vi "WildBugChilGru_V0.191.vi"() -> ()   [LabVIEW 2014]
uses:
  <vilib>/Utility/miscctls.llb/LVPointTypeDef.ctl
  <vilib>/Utility/xml.llb/Read From XML File(string).vi
  <vilib>/Utility/NIReport.llb/Append Report Text (str wrap).vi
  <vilib>/Utility/xml.llb/Write to XML File(string).vi
  <vilib>/Instr/_visa.llb/VISA Configure Serial Port (Instr).vi
  <vilib>/Analysis/3filter.llb/IIR Filter (DBL).vi
  <vilib>/Utility/NIReport.llb/NI_report.lvclass
  <vilib>/Analysis/NI_AALBase.lvlib
  <vilib>/gmath/NI_Gmath.lvlib
  <vilib>/Analysis/NI_AALPro.lvlib
panel:
  in  "Registerkarte":T1(tab)
  in  "Gleitender Mittelwert":u8=35
  in  "Differenzenquotient":u8=12
  in  "Polynom":u8=15
  in  "n vom Gas [1/min]":dbl=5000.0
  in  "Zündung [Imp/U]":u8=5
  in  "Übersetzung ermitteln aus":T2(ring)
  in  "Getriebe [1:]":dbl=5.343
  in  "Reifenumfang [m]":dbl=1.222
  in  "Dauer [s]":dbl=5.0
  in  "nKuWe/nRolle":dbl=10.0
  in  "Rolle [Inkr/U]":u16=10
  in  "Rollenumfang [m]":dbl=0.613
  in  "Rollenträgheit [kgm²]":dbl=0.402
  in  "Lufttemperatur [°C]":dbl=20.0
  in  "Luftfeuchtigkeit [%]":dbl=50.0
  in  "Luftdruck [mbar]":dbl=1013.0
  in  "Messung":bool
  in  "Ende":bool
  out "Datenspeicher":T3
  out "COM-Fehlerrate":string="0 / 0,0%"
  in  "Konfiguration:":bool
  in  "Speichern":bool
  in  "Drucken":bool
  out "Pmax":string="0,0 PS"
  out "Ergebnis":string="0,0 PS bei 0 1/min   |   0,0 Nm bei 0 1/min   |   vmax: 2147483647 km/h\nDIN 70020 k =1,000 (20 °C, 50 %, 1013 mbar)\n20.11.2016 20:05 "
  in  "Fahrzeugdaten":string="Hier die Fahrzeugdaten eingeben"
  out "XY-Graph":cluster{dbl[], dbl[]}[](graph)
  out "Untersetzung\nermittelt":bool
  out "Untersetzung":dbl format="%#.2f"
  in  "Start [F1]":bool
  out "Füllstand Lesepuffer":u64(slide) scale=1.0..100.0
  out "Hinterrad\n[km/h]":dbl(knob) scale=0.0..150.0
  out "Welle\n[1/min]":cluster{dbl, dbl}(knob) scale=0.0..12000.0
  out "Lesepuffer":string="\n"
  in  "Serielle Schnittstelle":refnum<visa-resource-name>="COM6"
  out "Untersetzung-Graph":dbl(graph)=2.6802446808510636 caption="Untersetzung"
  # "1. n konstant halten\n2. START\n3. n weiter halten\n4. bei GO: Vollgas\n5. vom Gas gehen"
  # "Zündung\nRolle"
  # "Untersetzung aus:"
  # "Eingabe <> Messen"
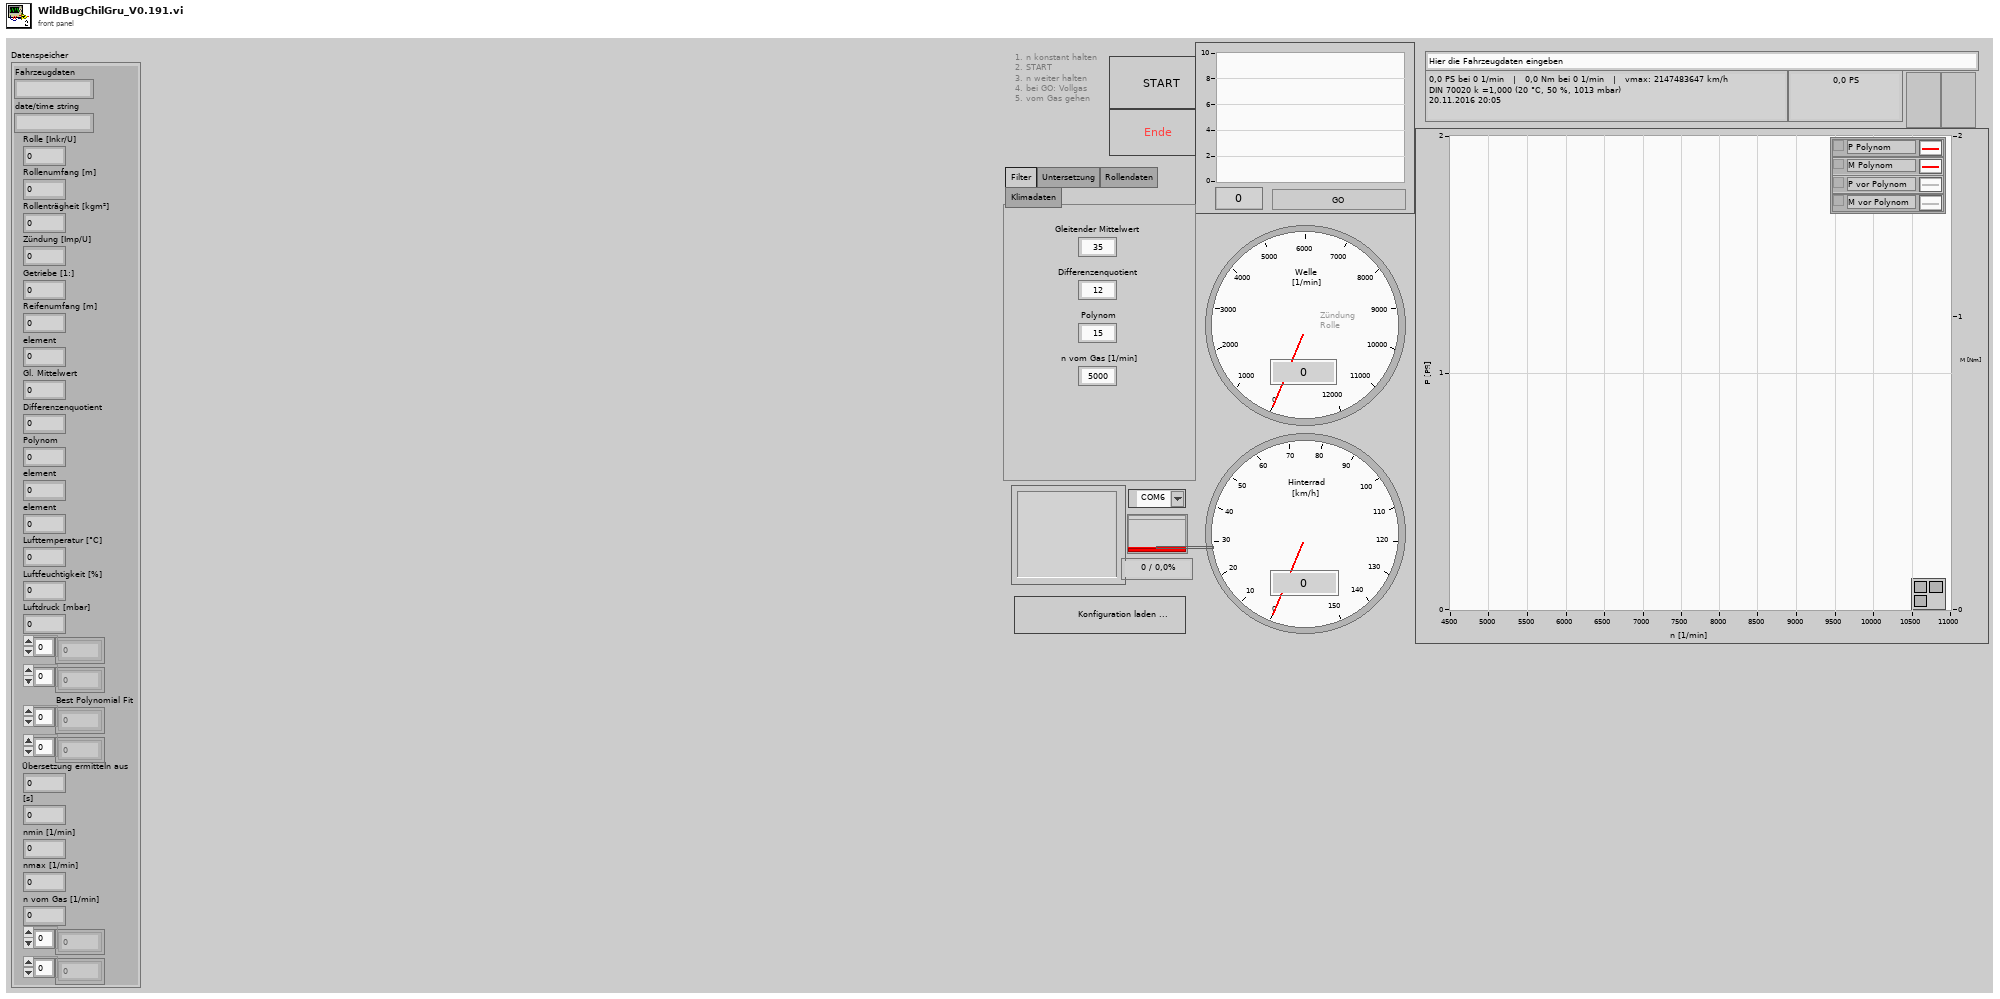
[diagram p1: front panel]
types:
  T1 = enum32{"Filter", "Untersetzung", "Rollendaten", "Klimadaten"}
  T2 = enum8{"Zündsignal", "Getriebe & Reifen", "nKuWe / nRolle"}
  T3 = cluster{"Fahrzeugdaten":string, "date/time string":string, "Rolle [Inkr/U]":u16, "Rollenumfang [m]":dbl, "Rollenträgheit [kgm²]":dbl, "Zündung [Imp/U]":u8, "Getriebe [1:]":dbl, "Reifenumfang [m] ":dbl, "element":dbl, "Gl. Mittelwert":u8, "Differenzenquotient":u8, "Polynom":u8, "element":dbl, "element":dbl, "Lufttemperatur [°C]":dbl, "Luftfeuchtigkeit [%]":dbl, "Luftdruck [mbar]":dbl, dbl[], dbl[], "Best Polynomial Fit":dbl[], dbl[], "Übersetzung ermitteln aus":u8, "[s]":dbl, "nmin [1/min]":dbl, "nmax [1/min]":dbl, "n vom Gas [1/min]":dbl, dbl[], i32[]}
  T4 = enum16{"Kleinste Quadrate", "Kleinestes absolutes Reiduum", "Biquadrat"}
  T5 = enum8{"Enabled", "Disabled", "Disabled and Grayed Out"}
  T6 = cluster{"Fahrzeugdaten":string, "date/time string":string, "Rolle [Inkr/U]":u16, "Rollenumfang [m]":dbl, "Rollenträgheit [kgm²]":dbl, "Zündung [Imp/U]":u8, "Getriebe [1:]":dbl, "Reifenumfang [m] ":dbl, "mean value":dbl, "Gleitender Mittelwert":u8, "Differenzenquotient":u8, "Polynom":u8, dbl, "element":dbl, "Lufttemperatur [°C]":dbl, "Luftfeuchtigkeit [%]":dbl, "Luftdruck [mbar]":dbl, dbl[], dbl[], "Best Polynomial Fit":dbl[], dbl[], "Übersetzung ermitteln aus":enum8{"Zündsignal", "Getriebe & Reifen", "nKuWe / nRolle"}, "Dauer [s]":dbl, dbl, dbl, "n vom Gas [1/min]":dbl, dbl[], i32[]}
  T7 = typedef "LVPointTypeDef.ctl" = cluster{"Horizontal":i16, "Vertical":i16}
  T8 = cluster{string, string, u16, dbl, dbl, u8, dbl, dbl, dbl, u8, u8, u8, dbl, dbl, dbl, dbl, dbl, dbl[], dbl[], dbl[], dbl[], i32, dbl, dbl, dbl, dbl, dbl[], i32[]}
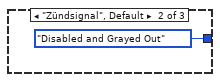
[diagram p2: hidden frame]
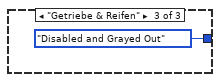
[diagram p3: hidden frame]
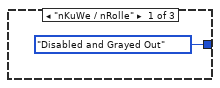
[diagram p4: hidden frame]
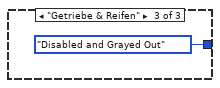
[diagram p5: hidden frame]
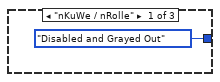
[diagram p6: hidden frame]
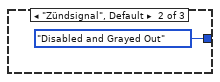
[diagram p7: hidden frame]
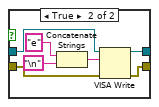
[diagram p11: hidden frame]
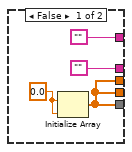
[diagram p13: hidden frame]
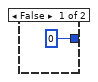
[diagram p14: hidden frame]
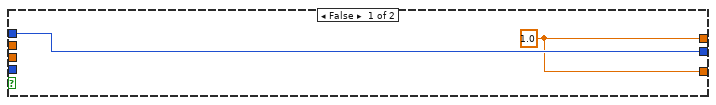
[diagram p16: hidden frame]
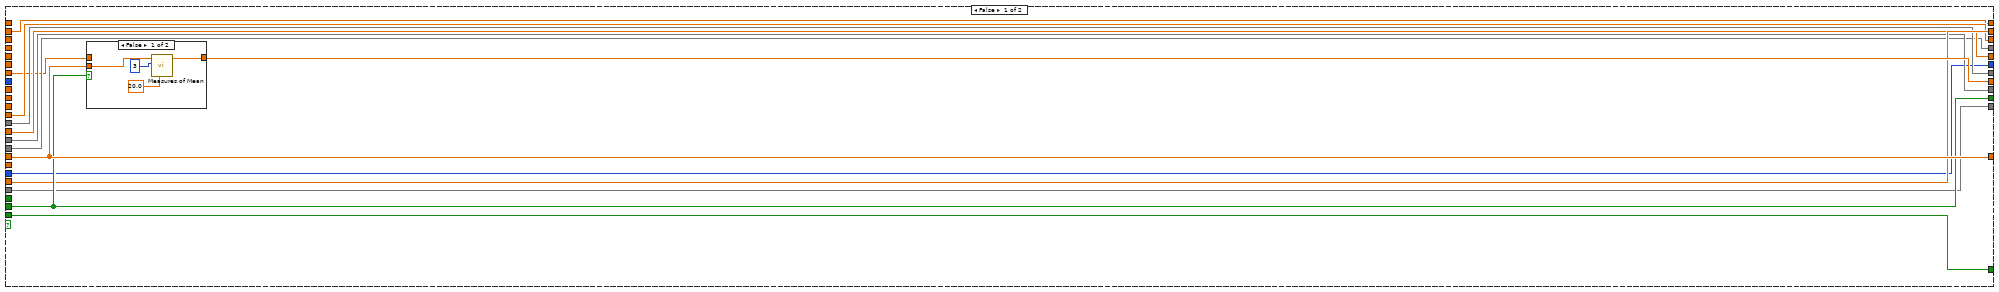
[diagram p17: hidden frame]
diagram:
  n1 = while {
    stop <- w1 stop-if-true
    n2 = event shown="[0] \"Start [F1]\": Wertänderung" {
      selector: _ -> [_ _]
      dyn-events: _ -> [_ _]
      timeout: _ -> [_ _]
      tunnel: [_ TRUE] -> w1
      event "Start [F1]": Value Change {
        n3 = event-data() -> ("NewVal"=w2:bool)  [unwired: 1 in, 5 out]
        n4 = case shown="True" w2 {
          frame False {
          }
          frame True {
            n5 = flat-sequence {
              tunnel: [w132] -> w117
              tunnel: [w131] -> w116
              tunnel: ["Messung"] -> w115
              tunnel: w117 -> [w145]
              tunnel: w116 -> [w144]
              tunnel: [0] -> w114
              tunnel: [1.0 ("element")] -> w113
              tunnel: [w142] -> w112
              tunnel: [w156] -> w111
              tunnel: [0] -> w110
              tunnel: [w142] -> w109
              tunnel: [-5] -> w108
              tunnel: [w153] -> w107
              tunnel: [w151] -> w106
              tunnel: [w150] -> w105
              tunnel: [0.0] -> w104
              tunnel: [w145] -> w103
              tunnel: [w144] -> w102
              tunnel: w115 -> [w143]
              tunnel: [w143] -> w101
              tunnel: w114 -> [w180]
              tunnel: [w180] -> w100
              tunnel: w113 -> [w179]
              tunnel: [w179] -> w99
              tunnel: w112 -> [w178]
              tunnel: [w178] -> w98
              tunnel: w111 -> [w177]
              tunnel: [w177] -> w97
              tunnel: w110 -> [w176]
              tunnel: [w176] -> w96
              tunnel: w109 -> [w175]
              tunnel: [w175] -> w95
              tunnel: w108 -> [w174]
              tunnel: [w174] -> w94
              tunnel: w107 -> [w173]
              tunnel: [w173] -> w93
              tunnel: w106 -> [w172]
              tunnel: [w172] -> w92
              tunnel: w105 -> [w171]
              tunnel: [w171] -> w91
              tunnel: w104 -> [w170]
              tunnel: [w170] -> w90
              tunnel: w103 -> [w169]
              tunnel: [w166] -> w89
              tunnel: w102 -> [w168]
              tunnel: [w167] -> w88
              tunnel: [w165] -> w87
              tunnel: w101 -> [w165]
              tunnel: w100 -> [w204]
              tunnel: [w204] -> w86
              tunnel: w99 -> [w203]
              tunnel: [w203] -> w85
              tunnel: w98 -> [w202]
              tunnel: [w202] -> w84
              tunnel: w97 -> [w201]
              tunnel: [w201] -> w83
              tunnel: w96 -> [w200]
              tunnel: [w200] -> w82
              tunnel: w95 -> [w199]
              tunnel: [w199] -> w81
              tunnel: w94 -> [w198]
              tunnel: [w198] -> w80
              tunnel: w93 -> [w197]
              tunnel: [w197] -> w79
              tunnel: w92 -> [w196]
              tunnel: [w196] -> w78
              tunnel: w91 -> [w195]
              tunnel: [w195] -> w77
              tunnel: w90 -> [w194]
              tunnel: [w194] -> w76
              tunnel: w89 -> [w193]
              tunnel: [w193] -> w75
              tunnel: w88 -> [w192]
              tunnel: [w192] -> w74
              tunnel: w87 -> [w190]
              tunnel: [w190] -> w73
              tunnel: w86 -> [w220]
              tunnel: [w220] -> w72
              tunnel: w85 -> [w219]
              tunnel: [w219] -> w71
              tunnel: w84 -> [w218]
              tunnel: [w218] -> w70
              tunnel: w83 -> [w217]
              tunnel: [w217] -> w69
              tunnel: w82 -> [w216]
              tunnel: [w216] -> w68
              tunnel: w81 -> [w215]
              tunnel: [w215] -> w67
              tunnel: w80 -> [w214]
              tunnel: [w214] -> w66
              tunnel: w79 -> [w213]
              tunnel: [w213] -> w65
              tunnel: w78 -> [w212]
              tunnel: [w212] -> w64
              tunnel: w77 -> [w211]
              tunnel: [w211] -> w63
              tunnel: w76 -> [w210]
              tunnel: [w210] -> w62
              tunnel: w75 -> [w209]
              tunnel: [w208] -> w61
              tunnel: w74 -> [w206]
              tunnel: [w207] -> w60
              tunnel: w73 -> [w205]
              tunnel: w72 -> [w293]
              tunnel: w71 -> [w292]
              tunnel: w70 -> [w291]
              tunnel: w69 -> [w290]
              tunnel: w68 -> [w289]
              tunnel: w67 -> [w288]
              tunnel: w66 -> [w287]
              tunnel: w65 -> [w286]
              tunnel: w64 -> [w285]
              tunnel: w63 -> [w284]
              tunnel: w62 -> [w283]
              tunnel: w61 -> [w248]
              tunnel: [w293] -> w59
              tunnel: [w292] -> w58
              tunnel: [w291] -> w57
              tunnel: [w290] -> w56
              tunnel: [w289] -> w55
              tunnel: [w288] -> w54
              tunnel: [w287] -> w53
              tunnel: [w286] -> w52
              tunnel: [w285] -> w51
              tunnel: [w284] -> w50
              tunnel: [w283] -> w49
              tunnel: [w248] -> w48
              tunnel: [w247] -> w47
              tunnel: [w282] -> w46
              tunnel: [w281] -> w45
              tunnel: [w280] -> w44
              tunnel: ["Gleitender Mittelwert"] -> w43
              tunnel: w60 -> [w247]
              tunnel: [w302] -> w9
              tunnel: [w303] -> w10
              tunnel: [w304] -> w11
              tunnel: [w305] -> w12
              tunnel: [w296] -> w7
              tunnel: [w295] -> w8
              tunnel: [w306] -> w13
              tunnel: [w307] -> w14
              tunnel: [w308] -> w16
              tunnel: [w309] -> w18
              tunnel: [w310] -> w19
              tunnel: [w311] -> w20
              tunnel: [w312] -> w37
              tunnel: [w313] -> w39
              tunnel: [w314] -> w40
              tunnel: [w315] -> w41
              tunnel: [w316] -> w42
              tunnel: w59 -> [w316]
              tunnel: w58 -> [w315]
              tunnel: w57 -> [w314]
              tunnel: w56 -> [w313]
              tunnel: w55 -> [w312]
              tunnel: w54 -> [w311]
              tunnel: w53 -> [w310]
              tunnel: w52 -> [w309]
              tunnel: w51 -> [w308]
              tunnel: w50 -> [w307]
              tunnel: w49 -> [w306]
              tunnel: w48 -> [w298]
              tunnel: w47 -> [w297]
              tunnel: w46 -> [w305]
              tunnel: w45 -> [w304]
              tunnel: w44 -> [w303]
              tunnel: w43 -> [w302]
              frame #0 {
                w137 = u16 0 items=["None", "XON/XOFF", "RTS/CTS", "XON/XOFF & RTS/CTS", "DTR/DSR", "XON/XOFF & DTR/DSR"] ("flow control (0:none)")
                w138 = u16 10 items=["1.0"=10, "1.5"=15, "2.0"=20] ("stop bits (10: 1 bit)")
                w130 = FALSE  # Enable Termination Char (T)
                w133 = u32 10000  # timeout (10sec)
                n6 = call-poly "VISA Configure Serial Port"("VISA resource name"="Serielle Schnittstelle", "timeout (10sec)"=w133, "Enable Termination\nChar (T)"=w130, "baud rate (9600)"=u32 250000 ("baudrate (250000)"), "data bits (8)"=u16 8, "parity (0:none)"=enum16{"None", "Odd", "Even", "Mark", "Space"}."None", "stop bits (10: 1 bit)"=w138, "flow control (0:none)"=w137) -> ("VISA resource name out"=w135:refnum<visa-resource-name>, "error out"=w134:errorcluster)  [unwired: 6 in]
                n7 = VISA Clear(VISA resource name=w135, error in (no error)=w134) -> (VISA resource name out=w132:refnum<visa-resource-name>, error out=w131:errorcluster)
              }
              frame #1 {
                w146 = T5."Disabled and Grayed Out" ("Deaktiviert")
                w149 = 0.0  # Graphen löschen
                w152 = 0
                w157 = 0.0
                w142 = FALSE
                w150 = ""
                n8 = case shown="True" w143 {
                  frame False {
                  }
                  frame True {
                    n9 = Wait (ms)(milliseconds to wait=u32 2000 ("Zu wartende ms")) -> ()  [unwired: 1 out]
                    n10 = property on="Untersetzung\nermittelt" class="Bool. (strikt)"("Blinking"=TRUE ("Blinkend"), "BoolText.Text"="Lese Klimadaten" ("Beschriftung.Text")) -> ()  [unwired: 2 in, 2 out]
                  }
                }
                n11 = Build Array(w149) -> (w148:dbl[])
                n12 = property on="Drucken" class="Bool. (strikt)"("DisabledEnum"=w146) -> ()  [unwired: 2 in, 2 out]
                n13 = property on="Übersetzung ermitteln aus" class="Enum (strikt)"("DisabledEnum"=w146) -> ()  [unwired: 2 in, 2 out]
                n14 = property on="Konfiguration:" class="Bool. (strikt)"("DisabledEnum"=w146) -> ()  [unwired: 2 in, 2 out]
                n15 = property on="Ende" class="Bool. (strikt)"("DisabledEnum"=w146) -> ()  [unwired: 2 in, 2 out]
                n16 = property on="Speichern" class="Bool. (strikt)"("DisabledEnum"=w146) -> ()  [unwired: 2 in, 2 out]
                n17 = local write "Pmax"(w150) -> ()
                n18 = property on="Untersetzung-Graph" class="SVDiagr (strikt)"("History Data"=w148) -> ()  [unwired: 2 in, 2 out]
                n19 = local write "COM-Fehlerrate"(w150) -> ()
                n20 = local write "Ergebnis"(w150) -> ()
                n21 = Initialize Array(0.0 ("y"), 0) -> (w153:dbl[])
                n22 = Initialize Array(w152, w152) -> (w151:i32[])
                n23 = Initialize Array(w157, w157) -> (w156:dbl[])
              }
              frame #2 {
                n24 = case shown="False" w165 {
                  tunnel: w169 -> [w182 w186]
                  tunnel: w168 -> [w181 w185]
                  tunnel: [w181 w184] -> w167
                  tunnel: [w182 w183] -> w166
                  frame False {
                  }
                  frame True {
                    n25 = Concatenate Strings("e" ("String"), "\n") -> (w189:string)
                    n26 = VISA Write(VISA resource name=w186, write buffer=w189, error in (no error)=w185) -> (VISA resource name out=w183:refnum<visa-resource-name>, error out=w184:errorcluster)  [unwired: 1 out]
                  }
                }
              }
              frame #3 {
                n27 = Wait (ms)(milliseconds to wait=u32 500 ("Zu wartende ms")) -> ()  [unwired: 1 out]
              }
              frame #4 {
                n28 = case shown="True" w205 {
                  tunnel: w209 -> [w222 w242]
                  tunnel: [w222 w241] -> w208
                  tunnel: [w221 w240] -> w207
                  tunnel: w206 -> [w221 w239]
                  frame False {
                  }
                  frame True {
                    w224 = ";" ("Regulärer Ausdruck")
                    n29 = property class="Instr"(reference=w242, error in=w239) -> (reference out=w245:refnum<visa-resource-name>, error out=w244:errorcluster, "Serial Settings:Number of Bytes at Serial Port"=w243:u32)
                    n30 = VISA Read(VISA resource name=w245, byte count=w243, error in (no error)=w244) -> (VISA resource name out=w241:refnum<visa-resource-name>, read buffer=w236:string, error out=w240:errorcluster)  [unwired: 1 out]
                    n31 = Search and Replace String(replace all?=TRUE ("Alle ersetzen? (F)"), input string=w236, search string="." ("Such-String"), replace string="," ("Ersetzungs-String (\"\")")) -> (result string=w229:string)  [unwired: 4 in, 3 out]
                    n32 = Match Pattern(string=w229, regular expression=w224) -> (before substring=w227:string, after substring=w228:string)  [unwired: 1 in, 2 out]
                    n33 = Fract/Exp String To Number(string=w227) -> (number=w235:dbl)  [unwired: 3 in, 1 out]
                    n34 = Match Pattern(string=w228, regular expression=w224) -> (before substring=w226:string, after substring=w225:string)  [unwired: 1 in, 2 out]
                    n35 = local write "Lufttemperatur [°C]"(w235) -> ()
                    n36 = Fract/Exp String To Number(string=w226) -> (number=w232:dbl)  [unwired: 3 in, 1 out]
                    n37 = Match Pattern(string=w225, regular expression=w224) -> (before substring=w223:string)  [unwired: 1 in, 3 out]
                    n38 = Fract/Exp String To Number(string=w223) -> (number=w234:dbl)  [unwired: 3 in, 1 out]
                    n39 = Divide(x=w232, y=100.0 ("x")) -> (x/y=w233:dbl)
                    n40 = local write "Luftdruck [mbar]"(w233) -> ()
                    n41 = local write "Luftfeuchtigkeit [%]"(w234) -> ()
                  }
                }
              }
              frame #5 {
                n42 = Wait (ms)(milliseconds to wait=u32 2000 ("Zu wartende ms")) -> ()  [unwired: 1 out]
                n43 = Add(x="Lufttemperatur [°C]", y=273.15) -> (x+y=w263:dbl)
                n44 = Divide ("M_Welle [Nm]")(x=300.0, y=w263) -> (x/y=w266:dbl)
                n45 = Multiply(x="Luftfeuchtigkeit [%]", y=0.01) -> (x*y=w277:dbl)
                n46 = Divide ("M_Welle [Nm]")(x=w263, y=293.15) -> (x/y=w261:dbl)
                n47 = Multiply(x=w277, y=240800000000.0) -> (x*y=w251:dbl)
                n48 = Power Of X(1:w266, 2:5.0) -> (0:w264:dbl)
                n49 = Multiply(x=w251, y=w264) -> (x*y=w271:dbl)
                n50 = Multiply(x=w266, y=-22.644) -> (x*y=w272:dbl)
                n51 = Power Of X(1:w261, 2:0.5) -> (0:w258:dbl)
                n52 = Exponential(1:w272) -> (0:w270:dbl)
                n53 = Multiply(x=w271, y=w270) -> (x*y=w269:dbl)
                n54 = Subtract "p_Trocken [mbar]"(x="Luftdruck [mbar]", y=w269) -> (x-y=w267:dbl)
                n55 = Divide ("M_Welle [Nm]")(x=1013.0, y=w267) -> (x/y=w259:dbl)
                n56 = Multiply "Korrekturfaktor DIN 70020"(x=w259, y=w258) -> (x*y=w282:dbl)
                n57 = Divide(x="Gleitender Mittelwert", y=2) -> (x/y=w255:dbl)
                n58 = Round Toward -Infinity(1:w255) -> (0:w254:dbl)
                n59 = call <vilib>:"Smoothing Filter Coefficients.vi"("shape"=1, "half-width"=w254, "type"=0) -> ("forward coefficients"=w280:dbl[], "reverse coefficients"=w281:dbl[])  [unwired: 6 in, 1 out]
              }
              frame #6 {
                n60 = Concatenate Strings("m" ("String"), "\n") -> (w301:string)
                n61 = property on="Untersetzung\nermittelt" class="Bool. (strikt)"("Blinking"=FALSE ("Blinkend")) -> ()  [unwired: 2 in, 2 out]
                n62 = VISA Write(VISA resource name=w298, write buffer=w301, error in (no error)=w297) -> (VISA resource name out=w295:refnum<visa-resource-name>, error out=w296:errorcluster)  [unwired: 1 out]
              }
            }
            n63 = while {
              tunnel: w8 -> [w447]
              tunnel: w7 -> [w446]
              shift-right: [w517] -> _
              shift-left: w14 -> [w462]
              shift-right: [w512] -> _
              shift-left: w13 -> [w516]
              shift-right: [w511] -> _
              shift-left: w13 -> [w515]
              shift-right: [w466] -> _
              shift-left: w13 -> [w514]
              shift-right: [w493] -> _
              shift-left: w42 -> [w513]
              shift-right: [w454] -> w25
              shift-left: w41 -> [_]
              shift-right: [w472] -> w29
              shift-left: w13 -> [w494]
              shift-right: [w504] -> w27
              shift-left: w13 -> [w468]
              shift-right: [w467] -> _
              shift-left: w18 -> [w508]
              shift-right: [w505] -> _
              shift-left: w40 -> [w482]
              shift-right: [w448] -> _
              shift-left: w39 -> [_]
              shift-right: [w453] -> _
              shift-left: w39 -> [_]
              shift-right: [w503] -> w28
              shift-left: w39 -> [w501]
              shift-right: [w502] -> _
              shift-left: w39 -> [w500]
              shift-right: [w488] -> w36
              shift-left: w18 -> [w499]
              shift-right: [w492] -> _
              shift-left: w18 -> [w497]
              shift-right: [w491] -> w32
              shift-left: w18 -> [w498]
              shift-right: [w490] -> w35
              shift-left: w18 -> [w496]
              shift-right: [w489] -> w34
              shift-left: w18 -> [w495]
              tunnel: [w487] -> w38
              shift-right: [w483] -> w33
              shift-left: w37 -> [w485]
              tunnel: [w486] -> w3
              tunnel: ["n vom Gas [1/min]"] -> w31
              tunnel: ["Rollenumfang [m]"] -> w30
              tunnel: ["Rollenumfang [m]"] -> w24
              shift-right: [w479] -> _
              shift-left: w20 -> [w445]
              shift-right: [w473] -> _
              shift-left: w19 -> [w478]
              shift-right: [w474] -> _
              shift-left: w13 -> [w477]
              shift-right: [w475] -> _
              shift-left: w13 -> [w476]
              shift-right: [w471] -> w17
              shift-left: w18 -> [w470]
              shift-right: [w465] -> _
              shift-left: _ -> [w464]
              shift-right: [w469] -> w15
              shift-left: w16 -> [w463]
              tunnel: [w461] -> w4
              tunnel: w12 -> [w454]
              tunnel: w11 -> [w448]
              tunnel: w10 -> [w453]
              tunnel: w9 -> [w452]
              stop <- w487 stop-if-true
              n64 = property class="Instr"(reference=w447, error in=w446) -> (reference out=w457:refnum<visa-resource-name>, error out=w456:errorcluster, "Serial Settings:Number of Bytes at Serial Port"=w459:u32)
              n65 = Greater?(x=w459, y=u32 1 ("min. Bytes")) -> (0:w455:bool)
              n66 = case shown="True" w455 {
                tunnel: w459 -> [_ w519]
                tunnel: [u32 0 ("Bytes at Port") w519] -> w458
                frame False {
                }
                frame True {
                }
              }
              n67 = case shown="1.." w458 {
                selector: w458 -> [_ w772]
                tunnel: [w722 w766] -> w486
                tunnel: [w721 w767] -> w461
                tunnel: [w726 w768] -> w511
                tunnel: [w727 w765] -> w512
                tunnel: w462 -> [w728 w763]
                tunnel: [w728 w761] -> w517
                tunnel: w516 -> [w727 w753]
                tunnel: w515 -> [w726 w752]
                tunnel: [w723 w751] -> w466
                tunnel: w514 -> [w723 w750]
                tunnel: w513 -> [w725 _]
                tunnel: [w725 w733] -> w493
                tunnel: [w724 w739] -> w465
                tunnel: w464 -> [w724 w738]
                tunnel: w457 -> [w721 w730]
                tunnel: w456 -> [w722 w729]
                frame 0, Default {
                  # "No data in from serial port - Nothing to do."
                }
                frame 1.. {
                  # "Hz Drum"
                  n68 = VISA Read(VISA resource name=w730, byte count=w772, error in (no error)=w729) -> (VISA resource name out=w767:refnum<visa-resource-name>, read buffer=w764:string, error out=w766:errorcluster)  [unwired: 1 out]
                  n69 = Concatenate Strings(w763, w764) -> (w735:string)
                  "Lesepuffer" <- w735
                  n70 = Spreadsheet String To Array(delimiter (Tab)="\n" ("regular expression"), format string="%s" ("regular expression"), spreadsheet string=w735, array type (2D Dbl)=string[] [] ("Array 2")) -> (array=w744:string[])
                  n71 = Match Pattern(string=w735, regular expression="[\\n]") -> (before substring=w742:string, after substring=w762:string, offset past match=w776:i32)  [unwired: 1 in, 1 out]
                  n72 = Array Size(array=w744) -> (size(s)=w748:i32)
                  n73 = Match Pattern(string=w742, regular expression="[;]") -> (before substring=w740:string, after substring=w741:string, offset past match=w737:i32)  [unwired: 1 in, 1 out]
                  n74 = Subtract "aktuelle Zeilenanzahl"(x=w748, y=1) -> (x-y=w733:i32)
                  n75 = property on="Füllstand Lesepuffer" class="Schieber (strikt)"() -> ("Scale.Maximum"=w732:dbl)  [unwired: 2 in, 2 out]
                  n76 = Match Pattern(string=w741, regular expression="[;]") -> (before substring=w771:string, after substring=w774:string, offset past match=w759:i32)  [unwired: 1 in, 1 out]
                  n77 = Match Pattern(string=w774, regular expression="[;]") -> (before substring=w770:string, after substring=w769:string, offset past match=w757:i32)  [unwired: 1 in, 1 out]
                  n78 = Greater Or Equal To 0?(x=w737) -> (x >= 0?=w736:bool)
                  n79 = Greater?(x=w733, y=w732) -> (0:w734:bool)
                  n80 = Greater Or Equal To 0?(x=w757) -> (x >= 0?=w756:bool)
                  n81 = Greater Or Equal To 0?(x=w759) -> (x >= 0?=w758:bool)
                  n82 = Greater Or Equal To 0?(x=w776) -> (x >= 0?=w760:bool)
                  n83 = Select(t=w733, s=w734, f=w732) -> (s? t:f=w731:dbl)
                  n84 = Build Array(w760, w758, w736, w756) -> (w755:bool[])
                  n85 = property on="Füllstand Lesepuffer" class="Schieber (strikt)"("Scale.Maximum"=w731) -> ()  [unwired: 2 in, 2 out]
                  n86 = And Array Elements(Boolean array=w755) -> (logical AND=w754:bool)
                  n87 = case shown="True" w754 {
                    tunnel: w771 -> [_ w787]
                    tunnel: w770 -> [_ w792]
                    tunnel: w769 -> [_ w791]
                    tunnel: [w780 w790] -> w768
                    tunnel: [w781 w789] -> w765
                    tunnel: w762 -> [_ w788]
                    tunnel: [w782 w788] -> w761
                    tunnel: w735 -> [w782 _]
                    tunnel: w753 -> [w781 _]
                    tunnel: w752 -> [w780 _]
                    tunnel: [w779 w786] -> w751
                    tunnel: w750 -> [w779 _]
                    tunnel: w740 -> [_ w785]
                    tunnel: [w778 w783] -> w739
                    tunnel: w738 -> [w778 _]
                    frame False {
                    }
                    frame True {
                      # "Cyclecounter"
                      # "Hz ComLevel"
                      # "ComLevel\nLevel 10 =   6Hz \nLevel 5 =   12Hz \nLevel 4 =   15Hz\nLevel 3 =   20Hz\nLevel 2 =   33Hz\nLevel 1 =   62Hz"
                      # "Hz Drum"
                      # "Hz Engine"
                      # "t4m"
                      n88 = Fract/Exp String To Number(string=w785) -> (number=w784:dbl)  [unwired: 3 in, 1 out]
                      n89 = Fract/Exp String To Number(string=w791) -> (number=w790:dbl)  [unwired: 3 in, 1 out]
                      n90 = Fract/Exp String To Number(string=w787) -> (number=w786:dbl)  [unwired: 3 in, 1 out]
                      n91 = To Long Integer(number=w784) -> (32bit integer=w783:i32)
                      n92 = Fract/Exp String To Number(string=w792) -> (number=w789:dbl)  [unwired: 3 in, 1 out]
                    }
                  }
                }
              }
              "Füllstand Lesepuffer" <- w493
              n93 = Not Equal?(x=w464, y=w465) -> (x != y?=w449:bool)
              n94 = case shown="True" w449 {
                tunnel: w478 -> [w523 w534]
                tunnel: [w523 w546] -> w473
                tunnel: w477 -> [w522 w545]
                tunnel: [w522 w531] -> w474
                tunnel: w476 -> [w521 w544]
                tunnel: [w521 w532] -> w475
                tunnel: w465 -> [_ w530]
                tunnel: w463 -> [w520 w529]
                tunnel: [w520 w533] -> w469
                frame False {
                }
                frame True {
                  n95 = Build Array (concatenate)(w529, w530) -> (w533:i32[])
                  n96 = Greater Or Equal To 0?(x=w534) -> (x >= 0?=w535:bool)
                  n97 = case shown="True" w535 {
                    tunnel: [w547 w558] -> w531
                    tunnel: [w547 w559] -> w532
                    tunnel: [w548 w550] -> w546
                    tunnel: w545 -> [_ w552]
                    tunnel: w544 -> [_ w560]
                    tunnel: w530 -> [w548 w549]
                    tunnel: w534 -> [_ w550]
                    frame False {
                      w547 = 1.0
                    }
                    frame True {
                      w556 = 65536.0
                      n98 = Add(x=w550, y=w552) -> (x+y=w551:dbl)
                      n99 = Divide(x=w551, y=w556) -> (x/y=w561:dbl)
                      n100 = Increment(x=w560) -> (x+1=w559:dbl)
                      n101 = Round Toward -Infinity(1:w561) -> (0:w557:dbl)
                      n102 = Multiply(x=w557, y=w556) -> (x*y=w555:dbl)
                      n103 = Add(x=w555, y=w549) -> (x+y=w554:dbl)
                      n104 = Increment(x=w554) -> (x+1=w553:dbl)
                      n105 = Subtract(x=w553, y=w550) -> (x-y=w558:dbl)
                    }
                  }
                  n106 = Subtract(x=w531, y=w532) -> (x-y=w526:dbl)
                  n107 = Decrement(x=w526) -> (x-1=w525:dbl)
                  n108 = Max & Min(x=0, y=w525) -> (max(x,y)=w524:dbl)  [unwired: 1 out]
                  n109 = Divide(x=w524, y=w531) -> (x/y=w538:dbl)
                  n110 = Greater Than 0?(x=w524) -> (x > 0?=w528:bool)
                  n111 = Select(t=u32 16711680, s=w528, f=u32 0) -> (s? t:f=w539:u32)
                  n112 = Multiply(x=w538, y=100.0) -> (x*y=w536:dbl)
                  n113 = Format Into String(format string="%d / %.1f%%" ("Format-String"), w524, w536) -> (resulting string=→"COM-Fehlerrate":string)  [unwired: 2 in, 1 out]
                  n114 = property on="COM-Fehlerrate" class="Str"("Text.TextColor"=w539) -> ()  [unwired: 2 in, 2 out]
                }
              }
              n115 = case "Case-Struktur" shown="True" w449 {
                tunnel: w512 -> [w702 w713]
                tunnel: w511 -> [w701 w712]
                tunnel: [w702 w711] -> w510
                tunnel: [w701 w710] -> w509
                tunnel: w466 -> [_ w704]
                tunnel: w494 -> [w700 _]
                tunnel: [w700 w703] -> w472
                tunnel: w468 -> [_ w709]
                tunnel: "Rollenumfang [m]" -> [_ w708]
                frame False {
                }
                frame True {
                  w720 = 60.0 ("y")
                  n116 = Reciprocal "Abtastzeit [s]"(x=w704) -> (1/x=w703:dbl)
                  n117 = Divide "R [1/s]"(x=w712, y="Rolle [Inkr/U]") -> (x/y=w719:dbl)
                  n118 = Multiply "nR [1/min]"(x=w720, y=w719) -> (x*y=w710:dbl)
                  n119 = Divide(x=w713, y="Zündung [Imp/U]") -> (x/y=w716:dbl)
                  n120 = Multiply "nZ gemessen [1/min]"(x=w716, y=w720) -> (x*y=w711:dbl)
                  n121 = Multiply "nZ berechnet [1/min]"(x=w710, y=w709) -> (x*y=w718:dbl)
                  n122 = Multiply "[m/min]"(x=w710, y=w708) -> (x*y=w714:dbl)
                  n123 = Multiply "[km/h]"(x=w714, y=0.06) -> (x*y=→"Hinterrad\n[km/h]":dbl)
                  n124 = Bundle(w711, w718) -> (→"Welle\n[1/min]":cluster{dbl, dbl})  [unwired: 1 in]
                }
              }
              n125 = case shown="True" w449 {
                tunnel: w510 -> [_ w631]
                tunnel: w509 -> [_ w630]
                tunnel: "Rollenumfang [m]" -> [_ w634]
                tunnel: [w573 w600] -> w504
                tunnel: w468 -> [w562 w600]
                tunnel: w482 -> [w574 w638]
                tunnel: w508 -> [w575 w637]
                tunnel: [w574 w591] -> w505
                tunnel: [w575 w636] -> w467
                tunnel: w448 -> [_ w633]
                tunnel: w453 -> [_ w632]
                tunnel: [w572 w586] -> w503
                tunnel: [w571 w584] -> w502
                tunnel: w501 -> [w572 w629]
                tunnel: w500 -> [w571 _]
                tunnel: w452 -> [_ w582]
                tunnel: [w570 w606] -> w488
                tunnel: w499 -> [w570 _]
                tunnel: [w569 w621] -> w492
                tunnel: w497 -> [w569 _]
                tunnel: w494 -> [_ w619]
                tunnel: [w568 w607] -> w491
                tunnel: w498 -> [w568 _]
                tunnel: [w567 w623] -> w490
                tunnel: w496 -> [w567 _]
                tunnel: [w566 w622] -> w489
                tunnel: w495 -> [w566 _]
                tunnel: w454 -> [_ w611]
                tunnel: w485 -> [w565 w605]
                tunnel: "n vom Gas [1/min]" -> [_ w593]
                tunnel: [w565 w604] -> w483
                tunnel: w482 -> [_ w603]
                tunnel: w445 -> [w564 w599]
                tunnel: [w564 w598] -> w479
                tunnel: w472 -> [_ w597]
                tunnel: [w563 w596] -> w471
                tunnel: w470 -> [w563 w595]
                frame False {
                  n126 = case shown="False" w574 {
                    tunnel: w575 -> [w579 _]
                    tunnel: [w578 w580] -> w573
                    tunnel: w562 -> [_ w580]
                    frame False {
                      n127 = call <vilib>:"Measures of Mean.vi"("percent (trim)"=20.0, "type"=3, "x array"=w579) -> ("mean value"=w578:dbl)  [unwired: 7 in, 1 out]
                    }
                    frame True {
                    }
                  }
                }
                frame True {
                  w614 = 0.00135962  # [W] in [PS]
                  w625 = 0.10471975511965978  # 2*Pi/60
                  n128 = Build Array (concatenate) "akt. dT in Array einfügen"(w595, w597) -> (w596:dbl[])
                  n129 = Build Array (concatenate) "akt. Rollendrehzahl\nin Array einfügen"(w629, w630) -> (w586:dbl[])
                  n130 = local read "Übersetzung ermitteln aus"() -> (w581:T2)
                  n131 = Square(x=w600) -> (x^2=w624:dbl)
                  n132 = Divide(x="Rollenträgheit [kgm²]", y=w624) -> (x/y=w612:dbl)
                  n133 = Index Array(array=w586, index=1 ("Index")) -> (element=w589:dbl)
                  n134 = Multiply(x=w612, y=w611) -> (x*y=w610:dbl)
                  n135 = Initialize Array(w589, w582) -> (w588:dbl[])
                  n136 = case shown="\"Getriebe & Reifen\"" w581 {
                    tunnel: w631 -> [_ _ w699]
                    tunnel: w630 -> [_ _ w698]
                    tunnel: [w694 "nKuWe/nRolle" w697] -> w635
                    tunnel: w634 -> [w695 _ _]
                    frame "Getriebe & Reifen" {
                      n137 = Divide(x=w695, y="Reifenumfang [m]") -> (x/y=w693:dbl)
                      n138 = Multiply(x=w693, y="Getriebe [1:]") -> (x*y=w694:dbl)
                    }
                    frame "nKuWe / nRolle" {
                    }
                    frame "Zündsignal" {
                      n139 = Divide(x=w699, y=w698) -> (x/y=w697:dbl)
                    }
                  }
                  n140 = Insert Into Array(array=w586, index=0 ("Index"), new element=w588) -> (w585:dbl[])
                  n141 = call-poly <vilib>:"IIR Filter.vi"("Forward Coefficients"=w632, "Reverse Coefficients"=w633, "X"=w585) -> ("Filtered X"=w583:dbl[])  [unwired: 1 in, 1 out]
                  n142 = Array Subset(array=w583, index=w582) -> (w584:dbl[])  [unwired: 1 in]
                  n143 = Multiply(x=2.0, y=w619) -> (x*y=w618:dbl)
                  n144 = case shown="False" w638 {
                    selector: w638 -> [_ w690]
                    tunnel: w635 -> [w679 _]
                    tunnel: w637 -> [w681 w689]
                    tunnel: [w675 w690] -> w628
                    tunnel: [w680 w689] -> w636
                    tunnel: w599 -> [w678 w688]
                    tunnel: [w675 w688] -> w598
                    tunnel: w581 -> [w676 _]
                    frame False {
                      n145 = Build Array (concatenate)(w681, w679) -> (w680:dbl[])
                      n146 = case shown="\"Zündsignal\"" w676 {
                        tunnel: ["Dauer [s]" 0.0 ("Dauer [s]")] -> w677
                        frame "Zündsignal" {
                          n147 = property on="Untersetzung\nermittelt" class="Bool. (strikt)"("Blinking"=TRUE ("Blinkend"), "BoolText.Text"="Ermittle Übersetzung" ("Boolescher Text.Text")) -> ()  [unwired: 2 in, 2 out]
                        }
                        frame "Getriebe & Reifen", Default {
                        }
                      }
                      n148 = call "Verstrichene Zeit"("Time Target (s)"=w677, "Reset"=w678) -> ("Time has Elapsed"=w675:bool)  [unwired: 10 in, 7 out]
                      n149 = case shown="True" w675 {
                        frame False {
                        }
                        frame True {
                          n150 = property on="Untersetzung\nermittelt" class="Bool. (strikt)"("Blinking"=FALSE ("Blinkend"), "BoolText.Text"="Go" ("Boolescher Text.Text")) -> ()  [unwired: 2 in, 2 out]
                        }
                      }
                      "Untersetzung-Graph" <- w679
                    }
                    frame True {
                    }
                  }
                  n151 = Array Size "Array-Größe"(array=w584) -> (size(s)=w626:i32)
                  n152 = Multiply(x=w584, y=w600) -> (x*y=w606:dbl[])
                  n153 = Multiply(x=w606, y=w625) -> (x*y=w621:dbl[])
                  n154 = Greater?(x=w626, y=w582) -> (0:w627:bool)
                  n155 = And(x=w628, y=w627) -> (x .and. y?=w591:bool)
                  n156 = Array Size "Array-Größe"(array=w621) -> (size(s)=w609:i32)
                  n157 = Decrement(x=w609) -> (x-1=w608:i32)
                  n158 = Select(t=w593, s=w591, f=1000000.0) -> (s? t:f=w594:dbl)
                  n159 = Initialize Array(0.0 ("y"), 0) -> (w615:dbl[])
                  n160 = for {
                    N: w609 -> [_]
                    tunnel: "Differenzenquotient" -> [w650]
                    tunnel: w621 -> [w658]
                    tunnel: w608 -> [w649]
                    tunnel: w618 -> [w659]
                    shift-right: [w655] -> w607
                    shift-left: w615 -> [w656]
                    tunnel: w606 -> [w653] mode=indexing
                    tunnel: w605 -> [w641]
                    tunnel: w594 -> [w652]
                    tunnel: [w642] -> w604
                    tunnel: w603 -> [w639]
                    i -> [w643]
                    stop <- w640 stop-if-true
                    n161 = Subtract(x=w649, y=w650) -> (x-y=w651:i32)
                    n162 = Subtract(x=w643, y=w650) -> (x-y=w672:i32)
                    n163 = Add(x=w643, y=w650) -> (x+y=w666:i32)
                    n164 = Greater Or Equal?(x=w643, y=w650) -> (x >= y?=w646:bool)
                    n165 = Greater?(x=w653, y=w652) -> (0:w654:bool)
                    n166 = Max & Min(x=w649, y=w666) -> (min(x,y)=w667:i32)  [unwired: 1 out]
                    n167 = Max & Min(x=w672, y=0) -> (max(x,y)=w670:i32)  [unwired: 1 out]
                    n168 = Subtract(x=w667, y=w643) -> (x-y=w668:i32)
                    n169 = Less Or Equal?(x=w643, y=w651) -> (x <= y?=w647:bool)
                    n170 = Subtract(x=w643, y=w670) -> (x-y=w669:i32)
                    n171 = Max & Min(x=w669, y=w668) -> (min(x,y)=w660:i32)  [unwired: 1 out]
                    n172 = Add(x=w643, y=w660) -> (x+y=w665:i32)
                    n173 = Subtract(x=w643, y=w660) -> (x-y=w664:i32)
                    n174 = Multiply(x=w660, y=w659) -> (x*y=w657:dbl)
                    n175 = Index Array(array=w658, index=w665) -> (element=w662:dbl)
                    n176 = Index Array(array=w658, index=w664) -> (element=w663:dbl)
                    n177 = Subtract(x=w662, y=w663) -> (x-y=w661:dbl)
                    n178 = Divide(x=w661, y=w657) -> (x/y=w648:dbl)
                    n179 = Less Than 0?(x=w648) -> (x < 0?=w645:bool)
                    n180 = Less Or Equal To 0?(x=w641) -> (x <= 0?=w644:bool)
                    n181 = Build Array (concatenate)(w656, w648) -> (w655:dbl[])
                    n182 = Compound Arithmetic op=AND(w645, w654, w644, w646, w647, w639) -> (w640:bool)
                    n183 = case shown="True" w640 {
                      tunnel: w643 -> [_ w674]
                      tunnel: [w673 w674] -> w642
                      tunnel: w641 -> [w673 _]
                      frame False {
                      }
                      frame True {
                      }
                    }
                  }
                  n184 = Multiply(x=w607, y=w610) -> (x*y=w623:dbl[])
                  n185 = Multiply(x=w621, y=w623) -> (x*y=w613:dbl[])
                  n186 = Multiply(x=w614, y=w613) -> (x*y=w622:dbl[])
                }
              }
              "Untersetzung\nermittelt" <- w505
              n187 = local read "Start [F1]"() -> (w451:bool)
              n188 = Greater Than 0?(x=w483) -> (x > 0?=w484:bool)
              n189 = Not(x=w451) -> (.not. x?=w450:bool)
              n190 = Select(t=w504, s=w505, f=0.0) -> (s? t:f=→"Untersetzung":dbl)
              n191 = Or(x=w484, y=w450) -> (x .or. y?=w487:bool)
            }
            n192 = VISA Clear(VISA resource name=w4, error in (no error)=w3) -> (VISA resource name out=w5:refnum<visa-resource-name>, error out=w6:errorcluster)
            n193 = case shown="True" w38 {
              tunnel: w36 -> [_ w421]
              tunnel: w35 -> [_ w426]
              tunnel: w34 -> [_ w425]
              tunnel: w33 -> [_ w397]
              tunnel: w32 -> [_ w422]
              tunnel: w31 -> [_ w420]
              tunnel: w30 -> [_ w414]
              tunnel: w25 -> [_ w400]
              tunnel: ["" w399] -> w26
              tunnel: w27 -> [_ w398]
              tunnel: ["" w396] -> _
              tunnel: [w360 w373] -> w23
              tunnel: [w360 w372] -> w22
              tunnel: [w360 w371] -> w21
              frame False {
                w361 = 0.0
                n194 = Initialize Array(w361, w361) -> (w360:dbl[])
              }
              frame True {
                w385 = 735.498  # PS in W
                w391 = 0.10471975511965978  # w = (2 * Pi / 60) * n
                w395 = 0
                n195 = Array Subset "P"(array=w425, length=w397) -> (w417:dbl[])  [unwired: 1 in]
                n196 = Array Subset "M"(array=w426, length=w397) -> (w418:dbl[])  [unwired: 1 in]
                n197 = Array Subset "alpha"(array=w422, length=w397) -> (w423:dbl[])  [unwired: 1 in]
                n198 = Array Subset "n"(array=w421, length=w397) -> (w419:dbl[])  [unwired: 1 in]
                n199 = property on="Pmax" class="Str"("Text.FontSize"=48) -> ()  [unwired: 2 in, 2 out]
                n200 = property on="Ergebnis" class="Str"("Text.FontSize"=18) -> ()  [unwired: 2 in, 2 out]
                n201 = Array Size(array=w423) -> (size(s)=w424:i32)
                n202 = for {
                  N: w424 -> [w444]
                  tunnel: w422 -> [w441]
                  tunnel: w421 -> [w438]
                  tunnel: w420 -> [w435]
                  tunnel: [w433] -> w393
                  i -> [w439]
                  stop <- w434 stop-if-true
                  n203 = Decrement(x=w444) -> (x-1=w443:i32)
                  n204 = Subtract(x=w443, y=w439) -> (x-y=w433:i32)
                  n205 = Index Array(array=w441, index=w433) -> (element=w442:dbl)
                  n206 = Index Array(array=w438, index=w433) -> (element=w437:dbl)
                  n207 = Less?(x=w437, y=w435) -> (x < y?=w436:bool)
                  n208 = Less Or Equal To 0?(x=w442) -> (x <= 0?=w440:bool)
                  n209 = And(x=w440, y=w436) -> (x .and. y?=w434:bool)
                }
                n210 = Increment(x=w393) -> (x+1=w392:i32)
                n211 = Array Subset "P"(array=w417, index=w392) -> (w394:dbl[])  [unwired: 1 in]
                n212 = Array Subset "M"(array=w418, index=w392) -> (w390:dbl[])  [unwired: 1 in]
                n213 = Array Subset "n"(array=w419, index=w392) -> (w373:dbl[])  [unwired: 1 in]
                n214 = local write "Polynom"("Polynom") -> ()
                n215 = Array Max & Min "nmax [1/min]"(array=w373) -> (max value=w416:dbl)  [unwired: 3 out]
                n216 = Bundle(w373, w390) -> (w378:cluster{dbl[], dbl[]})  [unwired: 1 in]
                n217 = Bundle(w373, w394) -> (w377:cluster{dbl[], dbl[]})  [unwired: 1 in]
                n218 = Multiply(x=w373, y=w391) -> (x*y=w387:dbl[])
                n219 = Array Size(array=w373) -> (size(s)=w370:i32)
                n220 = call <vilib>:"General Polynomial Fit.vi"("Y"=w390, "polynomial order"="Polynom", "X"=w373, "method"=T4."Biquadrat" ("Methode"), "algorithm"=3) -> ("Best Polynomial Fit"=w372:dbl[])  [unwired: 7 in, 3 out]
                n221 = Bundle(w373, "Best Polynomial Fit"=w372) -> (w379:cluster{dbl[], "Best Polynomial Fit":dbl[]})  [unwired: 1 in]
                n222 = Multiply(x=w372, y=w387) -> (x*y=w386:dbl[])
                n223 = Multiply(x=w370, y=0.8) -> (x*y=w381:dbl)
                n224 = Multiply(x=w370, y=0.1) -> (x*y=w364:dbl)
                n225 = Array Subset "MPoly ohne die ersten\nund letzten paar %"(array=w372, index=w364, length=w381) -> (w375:dbl[])
                n226 = Array Subset "n ohne die ersten \nund letzten paar %"(array=w373, index=w364, length=w381) -> ()  [unwired: 1 out]
                n227 = Divide(x=w416, y=w398) -> (x/y=w415:dbl)
                n228 = Divide(x=w386, y=w385) -> (x/y=w371:dbl[])
                n229 = Array Subset "PPoly ohne die ersten\nund letzten paar %"(array=w371, index=w364, length=w381) -> (w376:dbl[])
                n230 = Bundle(w373, w371) -> (w380:cluster{dbl[], dbl[]})  [unwired: 1 in]
                n231 = Compound Arithmetic op=MULTIPLY "vmax"(w415, w414, 0.06) -> (w406:dbl)
                n232 = Array Max & Min "Mmax"(array=w375) -> (max value=w383:dbl, max index (indices)=w366:i32)  [unwired: 2 out]
                n233 = Add(x=w364, y=w366) -> (x+y=w365:dbl)
                n234 = Multiply(x=w383, y=1.8) -> (x*y=w427:dbl)
                n235 = Index Array "n(Mmax)"(array=w373, index=w365) -> (element=w407:dbl)
                n236 = Array Max & Min "Pmax"(array=w376) -> (max value=w384:dbl, max index (indices)=w368:i32)  [unwired: 2 out]
                n237 = local read "Luftfeuchtigkeit [%]"() -> (w410:dbl)
                n238 = local read "Lufttemperatur [°C]"() -> (w409:dbl)
                n239 = Add(x=w364, y=w368) -> (x+y=w367:dbl)
                n240 = Build Array(w380, w379, w377, w378) -> (→"XY-Graph":cluster{dbl[], "Best Polynomial Fit":dbl[]}[])
                n241 = local read "Luftdruck [mbar]"() -> (w411:dbl)
                n242 = Multiply(x=w384, y=1.2) -> (x*y=w428:dbl)
                n243 = property on="XY-Graph" class="XYGraph (strikt)"("ActYScl"=1, "YScale.Maximum"=w427, "YScale.Minimum"=w395) -> ()  [unwired: 2 in, 2 out]
                n244 = property on="XY-Graph" class="XYGraph (strikt)"("ActYScl"=w395, "YScale.Maximum"=w428, "YScale.Minimum"=w395) -> ()  [unwired: 2 in, 2 out]
                n245 = Index Array "n(Pmax)"(array=w373, index=w367) -> (element=w412:dbl)
                n246 = Format Into String(format string="%.1f PS" ("Format-String"), w384) -> (resulting string=→"Pmax":string)  [unwired: 2 in, 1 out]
                n247 = Format Date/Time String(time format string (%c)="%x %H:%M ") -> (date/time string=w399:string)  [unwired: 2 in]
                n248 = Format Into String(format string="%.1f PS bei %d 1/min   |   %.1f Nm bei %d 1/min   |   vmax: %d km/h\\nDIN 70020 k =%.3f (%d \\B0C, %d %%, %d mbar)\\n%s" ("Format-String"), w384, w412, w383, w407, w406, w400, w409, w410, w411, w399) -> (resulting string=w396:string)  [unwired: 2 in, 1 out]
                "Ergebnis" <- w396
              }
            }
            n249 = VISA Close(VISA resource name=w5, error in (no error)=w6) -> ()  [unwired: 1 out]
            n250 = flat-sequence {
              tunnel: w15 -> [w321]
              tunnel: w17 -> [w322]
              tunnel: w21 -> [w323]
              tunnel: w22 -> [w324]
              tunnel: w23 -> [w325]
              tunnel: w24 -> [w326]
              tunnel: w25 -> [w327]
              tunnel: w26 -> [w328]
              tunnel: w27 -> [w329]
              tunnel: w28 -> [w330]
              tunnel: w29 -> [w331]
              tunnel: [w331] -> w128
              tunnel: [w330] -> w127
              tunnel: [w329] -> w126
              tunnel: [w328] -> w125
              tunnel: [w327] -> w124
              tunnel: [w326] -> w123
              tunnel: [w325] -> w122
              tunnel: [w324] -> w121
              tunnel: [w323] -> w120
              tunnel: [w322] -> w119
              tunnel: [w321] -> w118
              tunnel: w128 -> [w359]
              tunnel: w127 -> [w358]
              tunnel: w126 -> [w357]
              tunnel: w125 -> [w356]
              tunnel: w124 -> [w355]
              tunnel: w123 -> [w354]
              tunnel: w122 -> [w353]
              tunnel: w121 -> [w352]
              tunnel: w120 -> [w351]
              tunnel: w119 -> [w350]
              tunnel: w118 -> [w349]
              frame #0 {
                w318 = FALSE ("Start [F1]")
                w320 = 0  # Aktivieren
                n251 = property on="Untersetzung\nermittelt" class="Bool. (strikt)"("BoolText.Text"="GO" ("Boolescher Text.Text"), "Blinking"=w318) -> ()  [unwired: 2 in, 2 out]
                n252 = property on="XY-Graph" class="XYGraph (strikt)"("YScale.ScaleFit"=u8 1 ("X-Achse.Achsenanpassung")) -> ()  [unwired: 2 in, 2 out]
                n253 = property on="Speichern" class="Bool. (strikt)"("DisabledEnum"=w320) -> ()  [unwired: 2 in, 2 out]
                n254 = property on="Übersetzung ermitteln aus" class="Enum (strikt)"("DisabledEnum"=w320) -> ()  [unwired: 2 in, 2 out]
                n255 = property on="Konfiguration:" class="Bool. (strikt)"("DisabledEnum"=w320) -> ()  [unwired: 2 in, 2 out]
                n256 = property on="Ende" class="Bool. (strikt)"("DisabledEnum"=w320) -> ()  [unwired: 2 in, 2 out]
                n257 = property on="Drucken" class="Bool. (strikt)"("DisabledEnum"=w320) -> ()  [unwired: 2 in, 2 out]
                n258 = local write "Untersetzung\nermittelt"(w318) -> ()
                n259 = local write "Start [F1]"(w318) -> ()
              }
              frame #1 {
                w333 = 0.0
                n260 = local read "Übersetzung ermitteln aus"() -> (w336:T2)
                n261 = local read "Rollenträgheit [kgm²]"() -> (w346:dbl)
                n262 = local read "Gleitender Mittelwert"() -> (w342:u8)
                n263 = local read "Luftfeuchtigkeit [%]"() -> (w338:dbl)
                n264 = local read "Differenzenquotient"() -> (w341:u8)
                n265 = local read "Lufttemperatur [°C]"() -> (w339:dbl)
                n266 = local read "Reifenumfang [m]"() -> (w343:dbl)
                n267 = local read "n vom Gas [1/min]"() -> (w334:dbl)
                n268 = local read "Zündung [Imp/U]"() -> (w345:u8)
                n269 = local read "Luftdruck [mbar]"() -> (w337:dbl)
                n270 = local read "Rolle [Inkr/U]"() -> (w347:u16)
                n271 = local read "Getriebe [1:]"() -> (w344:dbl)
                n272 = local read "Polynom"() -> (w340:u8)
                n273 = local read "Dauer [s]"() -> (w335:dbl)
                n274 = Bundle("Fahrzeugdaten"="Fahrzeugdaten", "date/time string"=w356, "Rolle [Inkr/U]"=w347, "Rollenumfang [m]"=w354, "Rollenträgheit [kgm²]"=w346, "Zündung [Imp/U]"=w345, "Getriebe [1:]"=w344, "Reifenumfang [m]"=w343, "mean value"=w357, "Gleitender Mittelwert"=w342, "Differenzenquotient"=w341, "Polynom"=w340, w359, "element"=w355, "Lufttemperatur [°C]"=w339, "Luftfeuchtigkeit [%]"=w338, "Luftdruck [mbar]"=w337, w358, w353, "Best Polynomial Fit"=w352, w351, "Übersetzung ermitteln aus"=w336, "Dauer [s]"=w335, w333, w333, "n vom Gas [1/min]"=w334, w350, w349) -> (→"Datenspeicher":T6)  [unwired: 1 in]
              }
            }
          }
        }
      }
      event "Ende": Value Change {
        n275 = event-data() -> ()  [unwired: 1 in, 6 out]
      }
    }
  }
  n276 = flat-sequence {
    frame #0 {
      w810 = 0
      w806 = u8 0
      w804 = 0.0
      w808 = 0.0
      w803 = ""
      w813 = 2  # Deaktivieren
      w815 = 0.0  # Graphen löschen
      n277 = Initialize Array(w804, w804) -> (w809:dbl[])
      n278 = Initialize Array(w810, w810) -> (w811:i32[])
      n279 = local read "Serielle Schnittstelle"() -> (w801:refnum<visa-resource-name>)
      n280 = property on="Füllstand Lesepuffer" class="Schieber (strikt)"("Scale.Maximum"=100) -> ()  [unwired: 2 in, 2 out]
      n281 = property on="Frontpanel-Position" class="Bereich"("Origin"=T7 {"Horizontal"=8, "Vertical"=6}) -> ()  [unwired: 2 in, 2 out]
      n282 = Bundle(w803, w803, u16 0, w808, w808, w806, w808, w808, w808, w806, w806, w806, w808, w808, w808, w808, w808, w809, w809, w809, w809, 0, w808, w808, w808, w808, w809, w811) -> (w802:T8)  [unwired: 1 in]
      n283 = property on="Drucken" class="Bool. (strikt)"("DisabledEnum"=w813) -> ()  [unwired: 2 in, 2 out]
      n284 = property on="Speichern" class="Bool. (strikt)"("DisabledEnum"=w813) -> ()  [unwired: 2 in, 2 out]
      n285 = local write "Datenspeicher"(w802) -> ()
      n286 = VISA Clear(VISA resource name=w801) -> (VISA resource name out=w800:refnum<visa-resource-name>, error out=w799:errorcluster)  [unwired: 1 in]
      n287 = Build Array(w815) -> (w814:dbl[])
      n288 = VISA Close(VISA resource name=w800, error in (no error)=w799) -> (error out=w798:errorcluster)
      n289 = case shown="\"Getriebe & Reifen\"" "Übersetzung ermitteln aus" {
        tunnel: [T5."Disabled and Grayed Out" ("Deaktiviert") T5."Disabled and Grayed Out" ("Deaktiviert") T5."Enabled" ("Deaktiviert")] -> w797
        frame "nKuWe / nRolle" {
        }
        frame "Zündsignal", Default {
        }
        frame "Getriebe & Reifen" {
        }
      }
      n290 = case shown="\"Zündsignal\", Standard" "Übersetzung ermitteln aus" {
        tunnel: [T5."Disabled and Grayed Out" ("Deaktiviert") T5."Enabled" ("Deaktiviert") T5."Disabled and Grayed Out" ("Deaktiviert")] -> w796
        frame "nKuWe / nRolle" {
        }
        frame "Zündsignal", Default {
        }
        frame "Getriebe & Reifen" {
        }
      }
      n291 = case shown="\"nKuWe / nRolle\"" "Übersetzung ermitteln aus" {
        tunnel: [T5."Enabled" ("Deaktiviert") T5."Disabled and Grayed Out" ("Deaktiviert") T5."Disabled and Grayed Out" ("Deaktiviert")] -> w795
        frame "nKuWe / nRolle" {
        }
        frame "Zündsignal", Default {
        }
        frame "Getriebe & Reifen" {
        }
      }
      n292 = property on="Untersetzung-Graph" class="SVDiagr (strikt)"("History Data"=w814) -> ()  [unwired: 2 in, 2 out]
      n293 = case shown="Fehler" w798 {
        frame No Error {
        }
        frame Error {
          n294 = property on="Start [F1]" class="Bool. (strikt)"("DisabledEnum"=T5."Disabled and Grayed Out" ("Deaktiviert")) -> ()  [unwired: 2 in, 2 out]
        }
      }
      n295 = property on="Getriebe [1:]" class="DigWert (strikt)"("DisabledEnum"=w797) -> ()  [unwired: 2 in, 2 out]
      n296 = property on="Reifenumfang [m]" class="DigWert (strikt)"("DisabledEnum"=w797) -> ()  [unwired: 2 in, 2 out]
      n297 = property on="Zündung [Imp/U]" class="DigWert (strikt)"("DisabledEnum"=w796) -> ()  [unwired: 2 in, 2 out]
      n298 = property on="nKuWe/nRolle" class="DigWert (strikt)"("DisabledEnum"=w795) -> ()  [unwired: 2 in, 2 out]
    }
  }
  n299 = while {
    stop <- w827 stop-if-true
    n300 = event shown="[6] \"Übersetzung ermitteln aus\": Wertänderung" {
      selector: _ -> [_ _ _ _ _ _ _]
      dyn-events: _ -> [_ _ _ _ _ _ _]
      timeout: _ -> [_ _ _ _ _ _ _]
      tunnel: [_ _ _ TRUE _ _ _] -> w827
      event "Konfiguration:": Value Change {
        n301 = event-data() -> ("OldVal"=w828:bool)  [unwired: 1 in, 5 out]
        n302 = flat-sequence {
          tunnel: [w831] -> w829
          tunnel: w828 -> [w831]
          tunnel: w829 -> [w855]
          frame #0 {
            n303 = call-poly <vilib>:"Read From XML File.vi"() -> ("error out"=w834:errorcluster, "XML Elements"=w835:string)  [unwired: 9 in, 1 out]
            n304 = Unbundle By Name(w834) -> ("status"=w832:bool)
            n305 = property on="Datenspeicher" class="Cluster (strikt)"() -> ("Value"=w830:T3)  [unwired: 2 in, 2 out]
            n306 = Not(x=w832) -> (.not. x?=w833:bool)
            n307 = case shown="True" w833 {
              tunnel: w835 -> [_ w854]
              tunnel: w830 -> [_ w853]
              frame False {
              }
              frame True {
                n308 = Unflatten From XML(xml string=w854, type=w853) -> (value=w852:T3)  [unwired: 1 in, 1 out]
                n309 = Unbundle(w852) -> ("Fahrzeugdaten"=w851:string, "Rolle [Inkr/U]"=w850:u16, "Rollenumfang [m]"=w849:dbl, "Rollenträgheit [kgm²]"=w848:dbl, "Zündung [Imp/U]"=w847:u8, "Getriebe [1:]"=w846:dbl, "Reifenumfang [m]"=w845:dbl, "Gl. Mittelwert"=w844:u8, "Differenzenquotient"=w843:u8, "Polynom"=w842:u8, "Lufttemperatur [°C]"=w841:dbl, "Luftfeuchtigkeit [%]"=w840:dbl, "Luftdruck [mbar]"=w839:dbl, "Übersetzung ermitteln aus"=w836:u8, "[s]"=w838:dbl, "n vom Gas [1/min]"=w837:dbl)  [unwired: 12 out]
                n310 = property on="Polynom" class="DigWert (strikt)"("Value"=w842) -> ()  [unwired: 2 in, 2 out]
                n311 = property on="Dauer [s]" class="DigWert (strikt)"("Value"=w838) -> ()  [unwired: 2 in, 2 out]
                n312 = property on="Fahrzeugdaten" class="Str"("Value"=w851) -> ()  [unwired: 2 in, 2 out]
                n313 = property on="Rolle [Inkr/U]" class="DigWert (strikt)"("Value"=w850) -> ()  [unwired: 2 in, 2 out]
                n314 = property on="Rollenumfang [m]" class="DigWert (strikt)"("Value"=w849) -> ()  [unwired: 2 in, 2 out]
                n315 = property on="Rollenträgheit [kgm²]" class="DigWert (strikt)"("Value"=w848) -> ()  [unwired: 2 in, 2 out]
                n316 = property on="Zündung [Imp/U]" class="DigWert (strikt)"("Value"=w847) -> ()  [unwired: 2 in, 2 out]
                n317 = property on="Getriebe [1:]" class="DigWert (strikt)"("Value"=w846) -> ()  [unwired: 2 in, 2 out]
                n318 = property on="Reifenumfang [m]" class="DigWert (strikt)"("Value"=w845) -> ()  [unwired: 2 in, 2 out]
                n319 = property on="Gleitender Mittelwert" class="DigWert (strikt)"("Value"=w844) -> ()  [unwired: 2 in, 2 out]
                n320 = property on="Differenzenquotient" class="DigWert (strikt)"("Value"=w843) -> ()  [unwired: 2 in, 2 out]
                n321 = property on="Lufttemperatur [°C]" class="DigWert (strikt)"("Value"=w841) -> ()  [unwired: 2 in, 2 out]
                n322 = property on="Luftfeuchtigkeit [%]" class="DigWert (strikt)"("Value"=w840) -> ()  [unwired: 2 in, 2 out]
                n323 = property on="Luftdruck [mbar]" class="DigWert (strikt)"("Value"=w839) -> ()  [unwired: 2 in, 2 out]
                n324 = property on="Übersetzung ermitteln aus" class="Enum (strikt)"("Value"=w836) -> ()  [unwired: 2 in, 2 out]
                n325 = property on="n vom Gas [1/min]" class="DigWert (strikt)"("Value"=w837) -> ()  [unwired: 2 in, 2 out]
              }
            }
          }
          frame #1 {
            n326 = property on="Konfiguration:" class="Bool. (strikt)"("Value"=w855) -> ()  [unwired: 2 in, 2 out]
          }
        }
      }
      event "Drucken": Value Change {
        n327 = event-data() -> ("OldVal"=w856:bool)  [unwired: 1 in, 5 out]
        n328 = flat-sequence {
          tunnel: [w858] -> w857
          tunnel: w856 -> [w858]
          tunnel: w857 -> [w875]
          frame #0 {
            n329 = control-ref of="XY-Graph"() -> (w866:refnum<vi>)
            n330 = call <vilib>:"New Report.vi"("report type"=enum16{"Standard Report", "HTML"}."Standard Report") -> ("report out"=w861:refnum<class "NI_report.lvclass">, "error out"=w862:errorcluster)  [unwired: 13 in]
            n331 = property on="Fahrzeugdaten" class="Str"() -> ("Value"=w860:string)  [unwired: 2 in, 2 out]
            n332 = call-dynamic "Append Control Image to Report.vi"("report in"=w861, "image depth"=24, "ctrl reference"=w866, "error in (no error)"=w862) -> ("report out"=w868:refnum<class "NI_report.lvclass">, "error out"=w867:errorcluster)  [unwired: 8 in, 2 out]
            n333 = call-poly <vilib>:"Append Report Text.vi"("report in"=w868, "text"=w860, "error in (no error)"=w867) -> ("report out"=w869:refnum<class "NI_report.lvclass">, "error out"=w870:errorcluster)  [unwired: 9 in, 2 out]
            n334 = property on="Ergebnis" class="Str"() -> ("Value"=w859:string)  [unwired: 2 in, 2 out]
            n335 = call-poly <vilib>:"Append Report Text.vi"("report in"=w869, "text"=w859, "append on new line? (F)"=TRUE, "error in (no error)"=w870) -> ("report out"=w871:refnum<class "NI_report.lvclass">, "error out"=w872:errorcluster)  [unwired: 8 in, 2 out]
            n336 = call-dynamic "Print Report.vi"("report in"=w871, "error in (no error)"=w872) -> ("report out"=w865:refnum<class "NI_report.lvclass">, "error out"=w864:errorcluster)  [unwired: 12 in]
            n337 = call-dynamic "Dispose Report.vi"("report in"=w865, "error in (no error)"=w864) -> ()  [unwired: 13 in, 1 out]
          }
          frame #1 {
            n338 = property on="Drucken" class="Bool. (strikt)"("Value"=w875) -> ()  [unwired: 2 in, 2 out]
          }
        }
      }
      event "Speichern": Value Change {
        n339 = event-data() -> ("OldVal"=w876:bool)  [unwired: 1 in, 5 out]
        n340 = local read "Datenspeicher"() -> (w877:T3)
        n341 = local write "Speichern"(w876) -> ()
        n342 = Flatten To XML(anything=w877) -> (xml string=w879:string)
        n343 = call-poly <vilib>:"Write to XML File.vi"("XML Input"=w879) -> ("error out"=w878:errorcluster)  [unwired: 8 in, 2 out]
        n344 = case shown="Kein Fehler" w878 {
          frame No Error {
          }
          frame Error {
          }
        }
      }
      event "Ende": Value Change {
        n345 = event-data() -> ("OldVal"=w880:bool)  [unwired: 1 in, 5 out]
        n346 = local write "Ende"(w880) -> ()
      }
      event "Serielle Schnittstelle": Value Change {
        n347 = event-data() -> ()  [unwired: 1 in, 6 out]
        n348 = property on="Start [F1]" class="Bool. (strikt)"("DisabledEnum"=T5."Enabled" ("Deaktiviert")) -> ()  [unwired: 2 in, 2 out]
      }
      event "Messung": Value Change {
        n349 = event-data() -> ("NewVal"=w883:bool)  [unwired: 1 in, 5 out]
        n350 = case shown="True" w883 {
          frame True {
            w884 = T5."Disabled and Grayed Out" ("Deaktiviert")
            n351 = property on="Lufttemperatur [°C]" class="DigWert (strikt)"("DisabledEnum"=w884) -> ()  [unwired: 2 in, 2 out]
            n352 = property on="Luftdruck [mbar]" class="DigWert (strikt)"("DisabledEnum"=w884) -> ()  [unwired: 2 in, 2 out]
            n353 = property on="Luftfeuchtigkeit [%]" class="DigWert (strikt)"("DisabledEnum"=w884) -> ()  [unwired: 2 in, 2 out]
          }
          frame False {
            w885 = T5."Enabled" ("Deaktiviert")
            n354 = property on="Lufttemperatur [°C]" class="DigWert (strikt)"("DisabledEnum"=w885) -> ()  [unwired: 2 in, 2 out]
            n355 = property on="Luftdruck [mbar]" class="DigWert (strikt)"("DisabledEnum"=w885) -> ()  [unwired: 2 in, 2 out]
            n356 = property on="Luftfeuchtigkeit [%]" class="DigWert (strikt)"("DisabledEnum"=w885) -> ()  [unwired: 2 in, 2 out]
          }
        }
      }
      event "Übersetzung ermitteln aus": Value Change {
        n357 = event-data() -> ("NewVal"=w887:T2)  [unwired: 1 in, 5 out]
        n358 = case shown="\"nKuWe / nRolle\"" w887 {
          tunnel: [T5."Disabled and Grayed Out" ("Deaktiviert") T5."Disabled and Grayed Out" ("Deaktiviert") T5."Enabled" ("Deaktiviert")] -> w889
          frame "nKuWe / nRolle" {
          }
          frame "Zündsignal", Default {
          }
          frame "Getriebe & Reifen" {
          }
        }
        n359 = case shown="\"Zündsignal\", Standard" w887 {
          tunnel: [T5."Enabled" ("Deaktiviert") T5."Disabled and Grayed Out" ("Deaktiviert") T5."Disabled and Grayed Out" ("Deaktiviert")] -> w888
          frame "nKuWe / nRolle" {
          }
          frame "Zündsignal", Default {
          }
          frame "Getriebe & Reifen" {
          }
        }
        n360 = case shown="\"Zündsignal\", Standard" w887 {
          tunnel: [T5."Disabled and Grayed Out" ("Deaktiviert") T5."Enabled" ("Deaktiviert") T5."Disabled and Grayed Out" ("Deaktiviert")] -> w886
          frame "nKuWe / nRolle" {
          }
          frame "Zündsignal", Default {
          }
          frame "Getriebe & Reifen" {
          }
        }
        n361 = property on="Getriebe [1:]" class="DigWert (strikt)"("DisabledEnum"=w889) -> ()  [unwired: 2 in, 2 out]
        n362 = property on="Reifenumfang [m]" class="DigWert (strikt)"("DisabledEnum"=w889) -> ()  [unwired: 2 in, 2 out]
        n363 = property on="nKuWe/nRolle" class="DigWert (strikt)"("DisabledEnum"=w888) -> ()  [unwired: 2 in, 2 out]
        n364 = property on="Dauer [s]" class="DigWert (strikt)"("DisabledEnum"=w886) -> ()  [unwired: 2 in, 2 out]
        n365 = property on="Zündung [Imp/U]" class="DigWert (strikt)"("DisabledEnum"=w886) -> ()  [unwired: 2 in, 2 out]
      }
    }
  }
